vi "NotifyIcon.vi"   [LabVIEW 2013]
uses:
  System.Windows.Forms
  System.Drawing
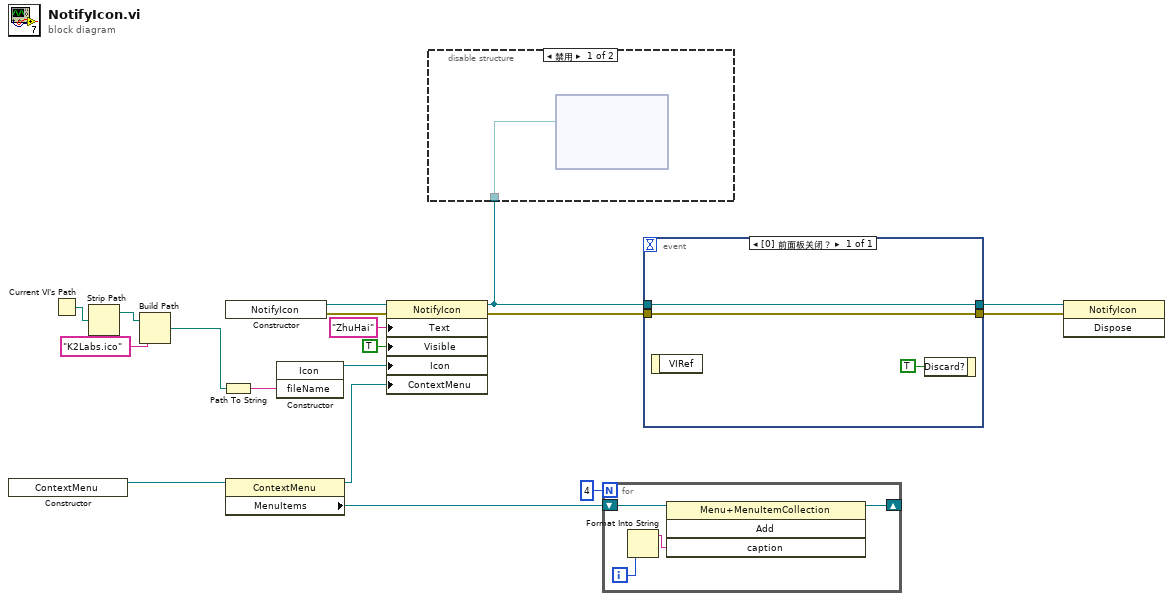
[diagram p0: block diagram]
diagram:
  n1 = constructor class="ContextMenu"() -> (reference out=w9:refnum<k24>)  [unwired: 3 in, 2 out]
  n2 = Current VI's Path() -> (path=w4:path)
  n3 = Strip Path(path=w4) -> (stripped path=w3:path)  [unwired: 1 out]
  n4 = Build Path(base path=w3, name or relative path="K2Labs.ico" ("名称或相对路径")) -> (appended path=w1:path)
  n5 = Path To String(path=w1) -> (string=w13:string)
  n6 = constructor class="NotifyIcon"() -> (reference out=w18:refnum<k24>, error out=w17:errorcluster)  [unwired: 3 in, 1 out]
  n7 = property class="ContextMenu"(reference=w9) -> (reference out=w8:refnum<k24>, "MenuItems"=w11:refnum<k24>)  [unwired: 1 in, 1 out]
  n8 = constructor class="Icon"("fileName"=w13) -> (reference out=w12:refnum<k24>)  [unwired: 3 in, 3 out]
  n9 = property class="NotifyIcon"(reference=w18, error in=w17, "Text"="ZhuHai", "Visible"=TRUE, "Icon"=w12, "ContextMenu"=w8) -> (reference out=w7:refnum<k24>, error out=w15:errorcluster)
  n10 = disable-structure shown="禁用" {
    disable-tunnel: w7 -> [w19 _]
    frame Disabled {
      n11 = node(w19) -> ()  [unwired: 4 in, 2 out]
    }
    frame Enabled {
    }
  }
  n12 = for {
    N: 4 -> [_]
    shift-right: [w22] -> _
    shift-left: w11 -> [w23]
    i -> [w21]
    n13 = Format Into String(w21) -> (resulting string=w20:string)  [unwired: 3 in, 1 out]
    n14 = invoke on="调用节点" class="Menu+MenuItemCollection" method="Add"(reference=w23, "caption"=w20) -> (reference out=w22:refnum<k24>)  [unwired: 2 in, 3 out]
  }
  n15 = event shown="[0] 前面板关闭？" {
    selector: _ -> [_]
    dyn-events: _ -> [_]
    timeout: _ -> [_]
    tunnel: w15 -> [w24]
    tunnel: w7 -> [w25]
    tunnel: [w25] -> w6
    tunnel: [w24] -> w5
    event Panel Close? {
      n16 = event-data() -> ()  [unwired: 1 in, 1 out]
      n17 = event-data("Discard?"=TRUE ("放弃？")) -> ()  [unwired: 1 in, 1 out]
    }
  }
  n18 = invoke on="调用节点" class="NotifyIcon" method="Dispose"(reference=w6, error in=w5) -> ()  [unwired: 1 in, 3 out]
